vi "Unflatten UIP Value.vi"(10 "String Value":string, 11 "Visible UIP In":refnum<class "VisibleUIP.lvclass">) -> (0 "Error Out":errorcluster, 3 "Visible UIP Out":refnum<class "VisibleUIP.lvclass">)   [LabVIEW 2020, in "UIM.lvlib" / "VisibleUIP.lvclass"]
uses:
  VisibleUIP.lvclass
  VisibleUIP.lvclass/VisibleUIP.ctl
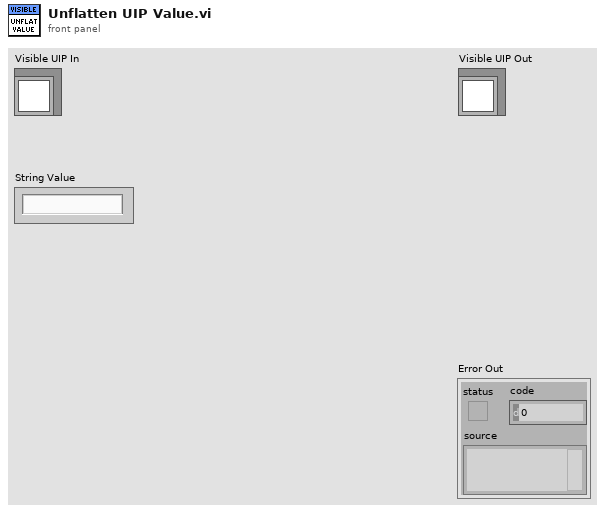
[diagram p1: front panel]
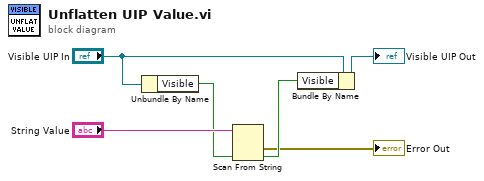
[diagram p0: block diagram]
diagram:
  n1 = Unbundle By Name("Visible UIP In") -> ("Visible"=w3:bool)
  n2 = Scan From String(input string="String Value", default 1=w3) -> (error out=→"Error Out":errorcluster, output 1=w2:bool)  [unwired: 3 in, 2 out]
  n3 = Bundle By Name(cluster="Visible UIP In", "Visible"=w2) -> (→"Visible UIP Out":refnum<class "VisibleUIP.lvclass">)
